vi "Get Stock Names.vi"() -> (3 "Stock Names":string[](array[string]))   [LabVIEW 2025, in "Full Featured MCP Server.lvlib"]
doc: "Returns the names of all stocks in same order as all other tools return the stocks."
uses:
  Full Featured MCP Server.lvlib
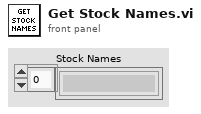
[diagram p1: front panel]
types:
  T1 = typedef "Full Featured MCP Server.lvlib/Server Data.ctl" = cluster{"Stocks Prices":dbl[][], "Owned Stocks":i32[], "Stock Names":string[], "Wallet":dbl, "Fluctuation":dbl, "Stock Trends":dbl[]}
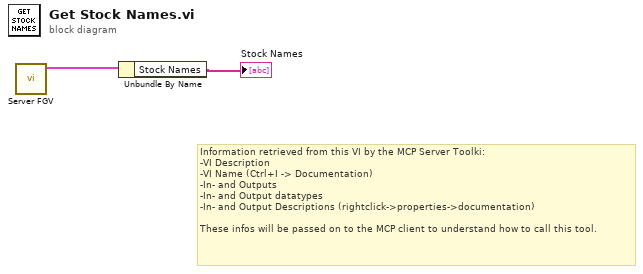
[diagram p0: block diagram]
diagram:
  # "Information retrieved from this VI by the MCP Server Toolki:\n-VI Description\n-VI Name (Ctrl+I -> Documentation)\n-In- and Outputs\n-In- and Output datatypes\n-In- and Output Descriptions (rightclick->properties->documentation)\n\nThese infos will be passed on to the MCP client to understand how to call this tool."
  n1 = call "Server FGV.vi"() -> ("Full Features MCP Server Data"=w1:T1)  [unwired: 9 in, 2 out]
  n2 = Unbundle By Name(w1) -> ("Stock Names"=→"Stock Names":string[])
